vi "writeSVs.vi"(8 "error in (no error)":errorcluster, 11 "ComponentData in":refnum<class "ComponentData.lvclass">) -> (0 "error out":errorcluster, 3 "ComponentData out":refnum<class "ComponentData.lvclass">)   [LabVIEW 2013, in "ComponentData.lvlib" / "ComponentData.lvclass"]
uses:
  <userlib>/Common/Component/common_application/RT/ComponentData/ComponentData/ComponentData.lvclass
  <userlib>/Common/Component/common_application/RT/ComponentData/ComponentData/ComponentData.lvclass/ComponentData.ctl
  <userlib>/Common/Component/common_application/RT/ComponentData/LoopTimer/LoopTimer.lvclass
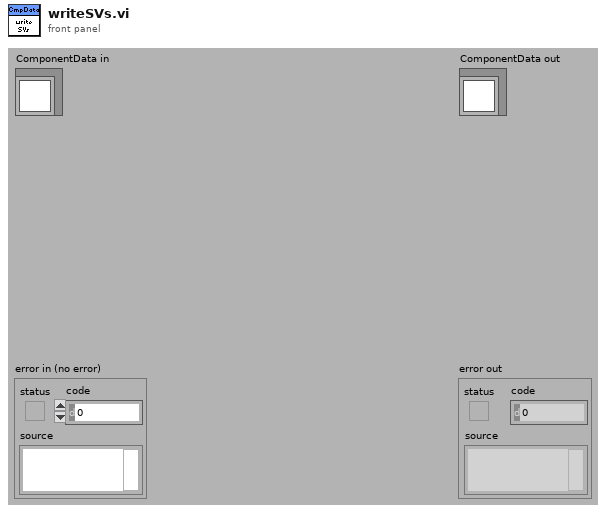
[diagram p1: front panel]
types:
  T1 = typedef "ComponentData.lvlib/componentStateValues.ctl" = enum16{"Off", "Standby", "Enabled", "Disabled", "Fault"}
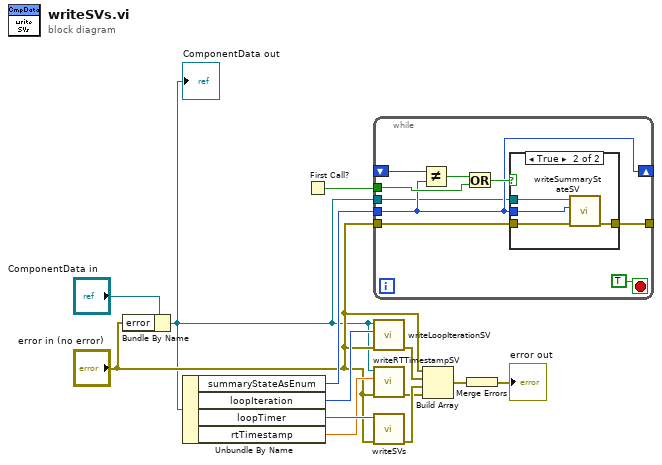
[diagram p0: block diagram]
diagram:
  n1 = Bundle By Name(cluster="ComponentData in", "error"="error in (no error)") -> (w1:refnum<class "ComponentData.lvclass">)
  "ComponentData out" <- w1
  n2 = Unbundle By Name(w1) -> ("summaryStateAsEnum"=w9:T1, "loopIteration"=w8:i32, "loopTimer"=w11:refnum<class "LoopTimer.lvclass">, "rtTimestamp"=w7:dbl)
  n3 = First Call?() -> (First Call?: T/F=w10:bool)
  n4 = while {
    shift-right: [w15] -> _
    shift-left: _ -> [w19]
    tunnel: w10 -> [w21]
    tunnel: [w17] -> _
    tunnel: "error in (no error)" -> [w16]
    tunnel: w9 -> [w15]
    tunnel: w1 -> [w14]
    stop <- TRUE stop-if-true
    n5 = Not Equal?(x=w19, y=w15) -> (x != y?=w20:bool)
    n6 = Or(x=w20, y=w21) -> (x .or. y?=w18:bool)
    n7 = case shown="True" w18 {
      tunnel: [w23 w25] -> w17
      tunnel: w16 -> [w23 w26]
      tunnel: w15 -> [_ w27]
      tunnel: w14 -> [_ w24]
      frame False {
      }
      frame True {
        n8 = call-dynamic "writeSummaryStateSV.vi"("error in (no error)"=w26, "componentStateValues"=w27, "ComponentData in"=w24) -> ("error out"=w25:errorcluster)  [unwired: 7 in, 1 out]
      }
    }
  }
  n9 = call-dynamic "writeLoopIterationSV.vi"("error in (no error)"="error in (no error)", "LoopIteration"=w8, "ComponentData in"=w1) -> ("error out"=w6:errorcluster)  [unwired: 7 in, 1 out]
  n10 = call-dynamic "writeRTTimestampSV.vi"("error in (no error)"="error in (no error)", "RTTimestamp"=w7, "ComponentData in"=w1) -> ("error out"=w4:errorcluster)  [unwired: 7 in, 1 out]
  n11 = call <userlib>:"writeSVs.vi"("error in (no error)"="error in (no error)", "LoopTimer in"=w11) -> ("error out"=w5:errorcluster)  [unwired: 8 in, 1 out]
  n12 = Build Array("error in (no error)", w6, w5, w4) -> (w12:errorcluster[])
  n13 = Merge Errors(w12) -> (→"error out":errorcluster)
